vi "byebyeMSG.vi"(1 "input":string, 2 "UDN":string, 3 "type of announce":u16(ring) items=["isRootDevice", "device", "service"]) -> (0 "byebyeMSG":string)   [LabVIEW 2010]
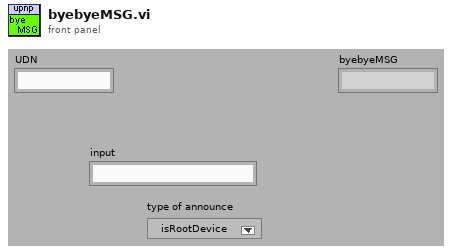
[diagram p1: front panel]
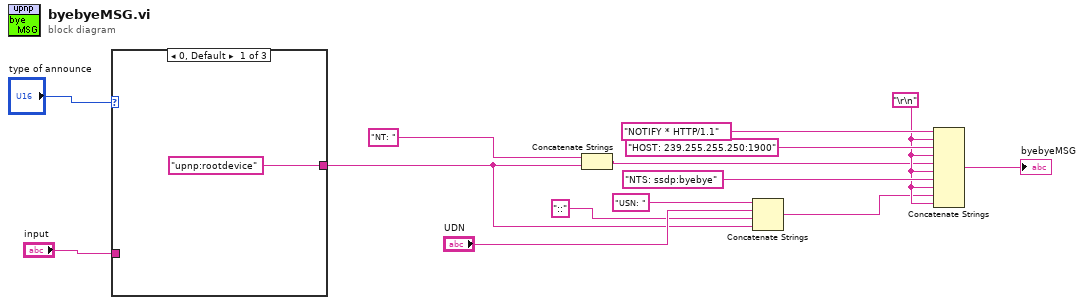
[diagram p0: block diagram]
diagram:
  w11 = "\r\n"
  n1 = case shown="0, Default" "type of announce" {
    tunnel: ["upnp:rootdevice" w16 w17] -> w1
    tunnel: "input" -> [_ w16 w17]
    frame 0, Default {
    }
    frame 1 {
    }
    frame 2 {
    }
  }
  n2 = Concatenate Strings("NT: " ("string"), w1) -> (w2:string)
  n3 = Concatenate Strings("USN: " ("string"), "UDN", "::" ("string"), w1) -> (w8:string)
  n4 = Concatenate Strings("NOTIFY * HTTP/1.1" ("string"), w11, "HOST: 239.255.255.250:1900" ("string"), w11, w2, w11, "NTS: ssdp:byebye" ("string"), w11, w8, w11) -> (→"byebyeMSG":string)
